vi "Enqueuer Global.vi"() -> ()   [LabVIEW 2020, in "Instrument Handler.lvlib" / "Instrument Handler.lvclass"]
doc: "This private global is used by the Instrument Handler to ensure that only one Instrument Handler is operational at a time."
uses:
  Instrument Handler.lvclass
  PPL/HDH.Actor Framework.Core.Actor.lvlibp/1abvi3w/vi.lib/ActorFramework/Message Enqueuer/Message Enqueuer.lvclass
panel:
  in  "Enqueuer":refnum<class "Message Enqueuer.lvclass">
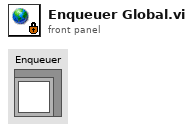
[diagram p1: front panel]
diagram:
